vi "CTL_BinarySearch.vi"(8 "Switched?":bool, 9 "PumpSpeed":enum16{"FAST", "SLOW", "CREEP", "STOP"}(ring), 10 "Spec Lo in":dbl, 11 "Spec HI in":dbl) -> (0 "Done":bool, 1 "Guess":dbl, 2 "Spec Lo out":dbl, 3 "Spec HI out":dbl)   [LabVIEW 2024]
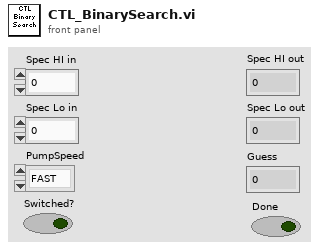
[diagram p1: front panel]
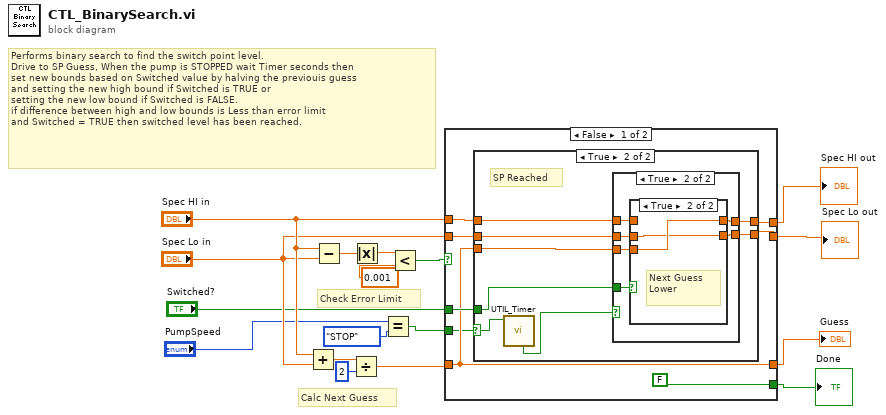
[diagram p0: block diagram]
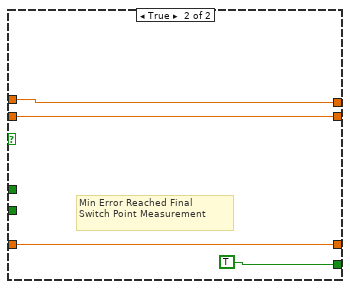
[diagram p5: hidden frame]
diagram:
  # "Performs binary search to find the switch point level.\nDrive to SP Guess, When the pump is STOPPED wait Timer seconds then \nset new bounds based on Switched value by halving the previouis guess\nand setting the new high bound if Switched is TRUE or\nsetting the new low bound if Switched is FALSE.\nif difference between high and low bounds is Less than error limit \nand Switched = TRUE then switched level has been reached."
  # "Check Error Limit"
  # "Calc Next Guess"
  n1 = Add(x="Spec HI in", y="Spec Lo in") -> (x+y=w5:dbl)
  n2 = Subtract(x="Spec HI in", y="Spec Lo in") -> (x-y=w7:dbl)
  n3 = Divide(x=w5, y=2) -> (x/y=w14:dbl)
  n4 = Absolute Value(x=w7) -> (abs(x)=w8:dbl)
  n5 = Equal?(x="PumpSpeed", y=enum16{"FAST", "SLOW", "CREEP", "STOP"}."STOP") -> (x = y?=w2:bool)
  n6 = Less?(x=w8, y=0.001) -> (x < y?=w10:bool)
  n7 = case shown="False" w10 {
    tunnel: "Spec Lo in" -> [w21 w50]
    tunnel: "Spec HI in" -> [w22 w49]
    tunnel: [FALSE TRUE] -> w11
    tunnel: "Switched?" -> [w24 _]
    tunnel: [w23 w50] -> w15
    tunnel: w14 -> [w19 w48]
    tunnel: [w20 w49] -> w17
    tunnel: [w19 w48] -> w4
    tunnel: w2 -> [w18 _]
    frame False {
      n8 = case shown="True" w18 {
        selector: w18 -> [_ w30]
        tunnel: w24 -> [_ w28]
        tunnel: [w26 w35] -> w23
        tunnel: w22 -> [w27 w34]
        tunnel: w21 -> [w26 w33]
        tunnel: [w27 w32] -> w20
        tunnel: w19 -> [_ w31]
        frame False {
          # "Waiting to Reach Set Point"
        }
        frame True {
          # "SP Reached"
          n9 = call "UTIL_Timer.vi"("Start"=w30) -> ("TO Trig"=w29:bool)  [unwired: 6 in, 4 out]
          n10 = case shown="True" w29 {
            tunnel: [w36 w43] -> w35
            tunnel: w34 -> [w37 w42]
            tunnel: w33 -> [w36 w41]
            tunnel: [w37 w40] -> w32
            tunnel: w31 -> [_ w39]
            tunnel: w28 -> [_ w38]
            frame False {
              # "Waiting for \nTimer to Expire"
            }
            frame True {
              n11 = case shown="True" w38 {
                tunnel: [w45 w46] -> w43
                tunnel: w39 -> [w45 w47]
                tunnel: w42 -> [w44 _]
                tunnel: w41 -> [_ w46]
                tunnel: [w44 w47] -> w40
                frame False {
                  # "Next Guess \nHigher"
                }
                frame True {
                  # "Next Guess \nLower"
                }
              }
            }
          }
        }
      }
    }
    frame True {
      # "Min Error Reached Final \nSwitch Point Measurement"
    }
  }
  "Guess" <- w4
  "Spec HI out" <- w17
  "Spec Lo out" <- w15
  "Done" <- w11
